vi "Puzzle 6.vi"() -> ()   [LabVIEW 2022 SP3]
panel:
  in  "delimited string":string="Time:        53     71     78     80\nDistance:   275   1181   1215   1524"
  out "size(s)":i32
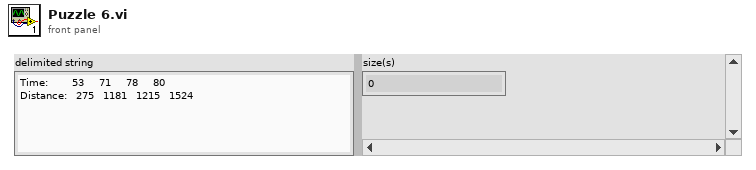
[diagram p1: front panel]
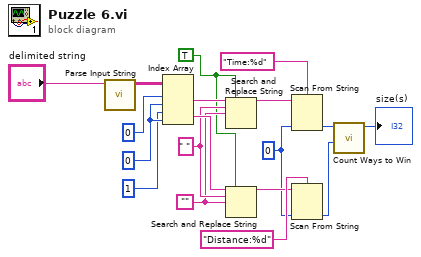
[diagram p0: block diagram]
diagram:
  w1 = i64 0 ("default value 1")
  w6 = "" ("replace string (\"\")")
  w5 = TRUE ("replace all? (F)")
  w7 = " " ("search string")
  w15 = 0 ("disabled index (col)")
  n1 = call "Parse Input String.vi"("delimited string"="delimited string") -> ("parsed string"=w17:string[][])  [unwired: 10 in]
  n2 = Index Array(array=w17, index (row) #1=0 ("disabled index (row)"), index (col) #1=w15, index (row) #2=1 ("disabled index (row)"), index (col) #2=w15) -> (element #1=w11:string, element #2=w9:string)
  n3 = Search and Replace String(replace all?=w5, input string=w11, search string=w7, replace string=w6) -> (result string=w10:string)  [unwired: 4 in, 3 out]
  n4 = Search and Replace String(replace all?=w5, input string=w9, search string=w7, replace string=w6) -> (result string=w8:string)  [unwired: 4 in, 3 out]
  n5 = Scan From String(format string="Time:%d", input string=w10, default 1=w1) -> (output 1=w4:i64)  [unwired: 2 in, 3 out]
  n6 = Scan From String(format string="Distance:%d", input string=w8, default 1=w1) -> (output 1=w3:i64)  [unwired: 2 in, 3 out]
  n7 = call "Count Ways to Win.vi"("previous record"=w3, "time"=w4) -> ("wins"=→"size(s)":i32)  [unwired: 9 in]
